vi "VBA处理模板.vi"(11 "NI_report输入":refnum<class "NI_report.lvclass">) -> (0 "错误输出":errorcluster)   [LabVIEW 2015]
uses:
  <vilib>/Utility/NIReport.llb/NI_report.lvclass
  Global.vi
  <vilib>/Utility/NIReport.llb/Excel/NI_Excel.lvclass
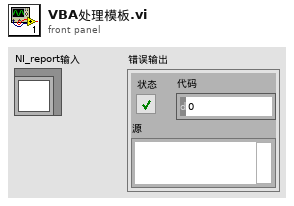
[diagram p1: front panel]
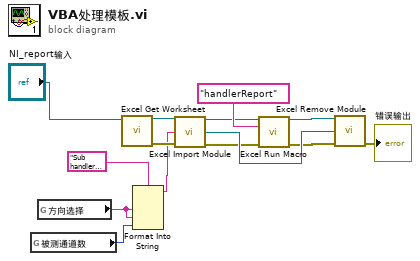
[diagram p0: block diagram]
diagram:
  n1 = global read "Global.vi" "被测通道数"() -> (w5:i32)
  n2 = global read "Global.vi" "方向选择"() -> (w4:string)
  n3 = call <vilib>:"Excel Get Worksheet.vi"("report in"="NI_report输入") -> ("report out"=w12:refnum<class "NI_report.lvclass">, "error out"=w13:errorcluster)  [unwired: 13 in]
  n4 = Format Into String(format string="Sub handlerReport()\n    Dim count As Integer\n    Dim col As String\n    Dim cuRange As String\n    Sheets(\"%S\").Select\n    '幅频响应\n    count = Sheets(\"测量点数\").Range(\"B2\")\n    If count <= 6 Then\n        Rows(\"16:27\").Hidden = True\n        col = CNtoW(count + 2)\n        cuRange = col & (10) & \":H\" & (15)\n        Range(cuRange).ClearContents\n    ElseIf count <= 12 Then\n        Rows(\"22:27\").Hidden = True\n        col = CNtoW(count - 6 + 2)\n        cuRange = col & (16) & \":H\" & (21)\n        Range(cuRange).ClearContents\n    ElseIf count <= 16 Then\n        col = CNtoW(count - 12 + 2)\n        cuRange = col & (22) & \":H\" & (27)\n        Range(cuRange).ClearContents\n    Else\n    End If\n    Call hideAmpborder(count, cuRange)\n    '幅值线性度\n    count = Sheets(\"测量点数\").Range(\"B3\")\n    If count <= 5 Then\n        Rows(\"35:40\").Hidden = True\n        col = CNtoW(count + 2)\n        cuRange = col & (29) & \":H\" & (34)\n        Range(cuRange).ClearContents\n    ElseIf count <= 10 Then\n        col = CNtoW(count - 5 + 2)\n        cuRange = col & (35) & \":H\" & (40)\n        Range(cuRange).ClearContents\n    Else\n    End If\n    Call hideLineborder(count, cuRange)\n    Call copyAndRemane(\"%S\", \"%d\")\nEnd Sub\n'列数转字母\nFunction CNtoW(ByVal num As Long) As String\n    CNtoW = Replace(Cells(1, num).Address(False, False), \"1\", \"\")\nEnd Function\n'隐藏边框(幅频响应)\nFunction hideAmpborder(ByVal hideCount As Integer, ByVal hideRange As String)\n    If hideCount <= 6 Then\n        Range(hideRange).Select\n        Selection.Borders(xlEdgeTop).LineStyle = xlNone\n        Selection.Borders(xlEdgeBottom).LineStyle = xlNone\n        Selection.Borders(xlEdgeRight).LineStyle = xlNone\n        Selection.Borders(xlInsideVertical).LineStyle = xlNone\n        Selection.Borders(xlInsideHorizontal).LineStyle = xlNone\n    ElseIf hideCount <= 16 Then\n        Range(hideRange).Select\n        Selection.Borders(xlEdgeBottom).LineStyle = xlNone\n        Selection.Borders(xlEdgeRight).LineStyle = xlNone\n        Selection.Borders(xlInsideVertical).LineStyle = xlNone\n        Selection.Borders(xlInsideHorizontal).LineStyle = xlNone\n    End If\nEnd Function\n'隐藏边框(幅值线性度)\nFunction hideLineborder(ByVal hideCount As Integer, ByVal hideRange As String)\n    If hideCount <= 5 Then\n        Range(hideRange).Select\n        Selection.Borders(xlEdgeTop).LineStyle = xlNone\n        Selection.Borders(xlEdgeBottom).LineStyle = xlNone\n        Selection.Borders(xlEdgeRight).LineStyle = xlNone\n        Selection.Borders(xlInsideVertical).LineStyle = xlNone\n        Selection.Borders(xlInsideHorizontal).LineStyle = xlNone\n    ElseIf hideCount <= 10 Then\n        Range(hideRange).Select\n        Selection.Borders(xlEdgeBottom).LineStyle = xlNone\n        Selection.Borders(xlEdgeRight).LineStyle = xlNone\n        Selection.Borders(xlInsideVertical).LineStyle = xlNone\n        Selection.Borders(xlInsideHorizontal).LineStyle = xlNone\n    End If\nEnd Function\n'根据方向和通道数更新excel 2021/5/31\nFunction copyAndRemane(ByVal direction As String, ByVal Channelno As Integer)\n    If Channelno = 2 Then\n        Sheets(direction).Copy after:=Sheets(direction)\n    ElseIf Channelno = 3 Then\n        Sheets(direction).Copy after:=Sheets(direction)\n        Sheets(direction).Copy after:=Sheets(direction)\n    Else\n    End If\nEnd Function", w4, w4, w5) -> (resulting string=w1:string)  [unwired: 2 in, 1 out]
  n5 = call <vilib>:"Excel Import Module.vi"("report in"=w12, "module code (\"\")"=w1, "error in (no error)"=w13) -> ("report out"=w6:refnum<class "NI_report.lvclass">, "module reference"=w11:refnum<k7>, "error out"=w7:errorcluster)  [unwired: 10 in]
  n6 = call <vilib>:"Excel Run Macro.vi"("report in"=w6, "macro name"="handlerReport", "error in (no error)"=w7) -> ("report out"=w9:refnum<class "NI_report.lvclass">, "error out"=w10:errorcluster)  [unwired: 10 in, 1 out]
  n7 = call <vilib>:"Excel Remove Module.vi"("report in"=w9, "module reference"=w11, "error in (no error)"=w10) -> ("error out"=→"错误输出":errorcluster)  [unwired: 11 in, 1 out]
